vi "Enqueue - Multiple Clusters.vi"(5 "Insert? (T)":bool=TRUE, 7 "At Front?":bool, 8 "error in":errorcluster, 10 "Array of Clusters":T2[](array[typedef]), 11 "Queue with Cluster Reference":T1) -> (0 "error out":errorcluster, 3 "Queue (dup)":T1)   [LabVIEW 2010]
doc: "This VI enqueues mulitple command and data clusters into the referenced queue.\n\nInputs:\nQueue with Cluster Reference - (queue) queue to insert cluster into\nArray of Clusters - (cluster array) array of command/data cluster to insert into the queue\nAt Front? (F) - (bool) set TRUE to insert cluster at the beginning of the queue; FALSE (default) at the end\nInsert? (T) - (bool) TRUE = insert cluster into queue (default); FALSE = do not insert cluster (controlled via logic)\nerror in - error input cluster\n\nOutputs:\nQueue Out (dup) - (queue) duplicate reference to input queue\nerror out - error output cluster"
uses:
  <userlib>/Common/Queue with Cluster/TYP_Queue Cluster Element.ctl
  <userlib>/Common/Queue with Cluster/TYP_Queue with Cluster Reference.ctl
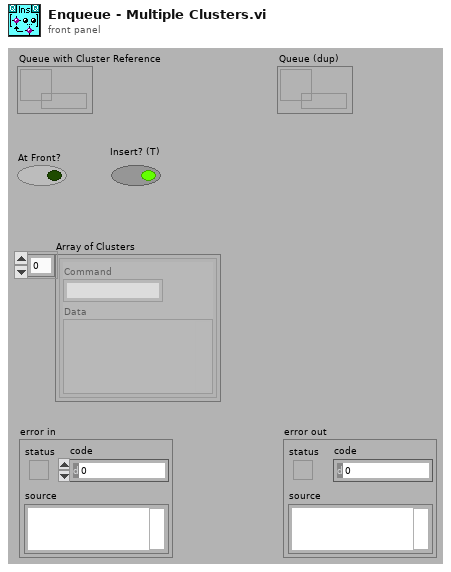
[diagram p1: front panel]
types:
  T1 = typedef "TYP_Queue with Cluster Reference.ctl" = refnum<queue>
  T2 = typedef "TYP_Queue Cluster Element.ctl" = cluster{"Command":string, "Data":variant}
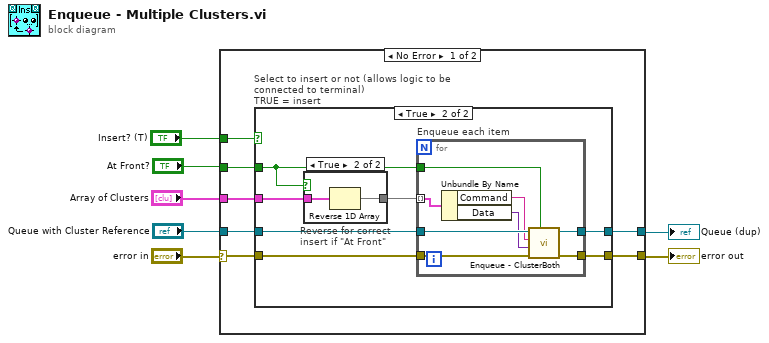
[diagram p0: block diagram]
diagram:
  n1 = case shown="No Error" "error in" {
    selector: "error in" -> [w11 w36]
    tunnel: "Array of Clusters" -> [w10 _]
    tunnel: "Queue with Cluster Reference" -> [w14 w35]
    tunnel: [w13 w35] -> w3
    tunnel: [w12 w36] -> w6
    tunnel: "At Front?" -> [w9 _]
    tunnel: "Insert? (T)" -> [w8 _]
    frame No Error {
      n2 = case "Select to insert or not (allows logic to be connected to terminal)\nTRUE = insert" shown="True" w8 {
        tunnel: w14 -> [w15 w23]
        tunnel: [w15 w22] -> w13
        tunnel: [w16 w21] -> w12
        tunnel: w11 -> [w16 w20]
        tunnel: w10 -> [_ w18]
        tunnel: w9 -> [_ w19]
        frame False {
        }
        frame True {
          n3 = case "Reverse for correct\ninsert if \"At Front\"" shown="True" w19 {
            tunnel: w18 -> [w24 w26]
            tunnel: [w24 w25] -> w17
            frame False {
            }
            frame True {
              n4 = Reverse 1D Array(array=w26) -> (reversed array=w25:T2[])
            }
          }
          n5 = for "Enqueue each item" {
            tunnel: w23 -> [w31]
            tunnel: w20 -> [w32]
            tunnel: [w34] -> w22
            tunnel: [w33] -> w21
            tunnel: w17 -> [w30] mode=indexing
            tunnel: w19 -> [w27]
            n6 = Unbundle By Name(w30) -> ("Command"=w28:string, "Data"=w29:variant)
            n7 = call "Enqueue - ClusterBoth.vi"("At Front? (F)"=w27, "error in (no error)"=w32, "Data"=w29, "Command"=w28, "Queue with Cluster Reference"=w31) -> ("error out"=w33:errorcluster, "Queue Out (dup)"=w34:T1)  [unwired: 5 in]
          }
        }
      }
    }
    frame Error {
    }
  }
  "error out" <- w6
  "Queue (dup)" <- w3
